vi "Auto Locate.vi"() -> (0 "Located":bool, 1 "zAvit":dbl, 2 "X Drive Arcade":dbl)   [LabVIEW 2012]
uses:
  BotStatus.vi
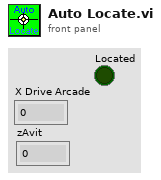
[diagram p1: front panel]
types:
  T1 = cluster{"Target Position X":dbl, "Target Position Y":dbl, "Center Target":bool}
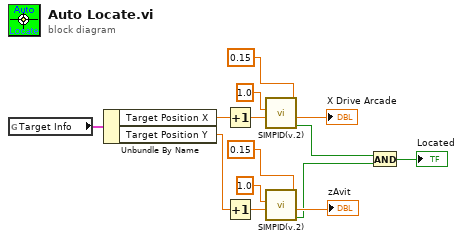
[diagram p0: block diagram]
diagram:
  n1 = global read "BotStatus.vi" "Target Info"() -> (w12:T1)
  n2 = Unbundle By Name(w12) -> ("Target Position X"=w7:dbl, "Target Position Y"=w11:dbl)
  n3 = Increment(x=w7) -> (x+1=w6:dbl)
  n4 = Increment(x=w11) -> (x+1=w10:dbl)
  n5 = call "SIMPID(v.2).vi"("Range"=0.15, "Current Point"=w6, "Set Point"=1.0) -> ("On Target"=w2:bool, "result"=→"X Drive Arcade":dbl)  [unwired: 7 in]
  n6 = call "SIMPID(v.2).vi"("Range"=0.15, "Current Point"=w10, "Set Point"=1.0) -> ("On Target"=w3:bool, "result"=→"zAvit":dbl)  [unwired: 7 in]
  n7 = And(x=w2, y=w3) -> (x .and. y?=→"Located":bool)
